vi "for_auto_sensitivity.vi"(6 "Sensutivity old":dbl, 8 "Ch4 percent":dbl, 9 "Ch3 percent":dbl, 10 "Ch2 percent":dbl, 11 "Ch1 percent":dbl) -> (2 "Sensitivity new":dbl, 3 "Change sensitivity":bool)   [LabVIEW 2019]
panel:
  out "Increase":bool
  out "Decrease":bool
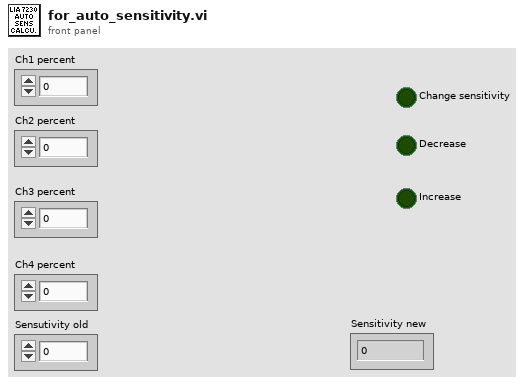
[diagram p1: front panel]
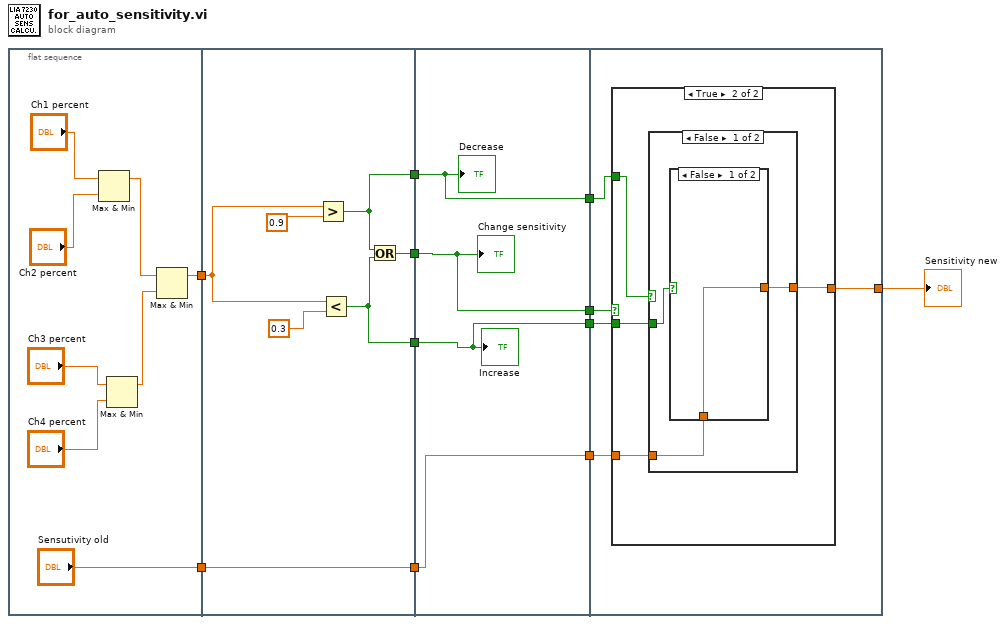
[diagram p0: block diagram]
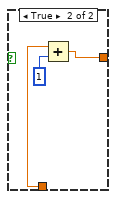
[diagram p3: hidden frame]
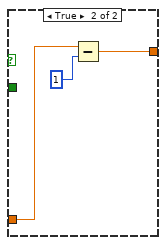
[diagram p4: hidden frame]
diagram:
  n1 = flat-sequence {
    tunnel: ["Sensutivity old"] -> w11
    tunnel: [w12] -> w9
    tunnel: w11 -> [w26]
    tunnel: [w26] -> w10
    tunnel: w9 -> [w25]
    tunnel: [w22] -> w8
    tunnel: [w21] -> w7
    tunnel: [w20] -> w6
    tunnel: w10 -> [w29]
    tunnel: w8 -> [w30]
    tunnel: w7 -> [w28]
    tunnel: w6 -> [w27]
    tunnel: [w30] -> w5
    tunnel: [w29] -> w4
    tunnel: [w28] -> w2
    tunnel: [w27] -> w1
    tunnel: w5 -> [w35]
    tunnel: w4 -> [w34]
    tunnel: [w33] -> w3
    tunnel: w2 -> [w32]
    tunnel: w1 -> [w31]
    frame #0 {
      n2 = Max & Min(x="Ch1 percent", y="Ch2 percent") -> (max(x,y)=w14:dbl)  [unwired: 1 out]
      n3 = Max & Min(x="Ch3 percent", y="Ch4 percent") -> (max(x,y)=w13:dbl)  [unwired: 1 out]
      n4 = Max & Min(x=w14, y=w13) -> (max(x,y)=w12:dbl)  [unwired: 1 out]
    }
    frame #1 {
      n5 = Greater?(x=w25, y=0.9) -> (0:w21:bool)
      n6 = Less?(x=w25, y=0.3) -> (x < y?=w20:bool)
      n7 = Or(x=w21, y=w20) -> (x .or. y?=w22:bool)
    }
    frame #2 {
      "Decrease" <- w28
      "Increase" <- w27
      "Change sensitivity" <- w30
    }
    frame #3 {
      n8 = case shown="True" w35 {
        tunnel: w34 -> [w36 w39]
        tunnel: [w36 w38] -> w33
        tunnel: w32 -> [_ w40]
        tunnel: w31 -> [_ w37]
        frame False {
        }
        frame True {
          n9 = case shown="False" w40 {
            tunnel: w39 -> [w42 w50]
            tunnel: [w41 w48] -> w38
            tunnel: w37 -> [w43 _]
            frame False {
              n10 = case shown="False" w43 {
                tunnel: w42 -> [w44 w47]
                tunnel: [w44 w45] -> w41
                frame False {
                }
                frame True {
                  n11 = Add(x=w47, y=1) -> (x+y=w45:dbl)
                }
              }
            }
            frame True {
              n12 = Subtract(x=w50, y=1) -> (x-y=w48:dbl)
            }
          }
        }
      }
    }
  }
  "Sensitivity new" <- w3
